vi "Tacking Helper - Jump Length.vi"(9 "Bounding box\nside length (m?)":dbl, 10 "Second\nArm Length":dbl, 11 "Starting\nArm Length":dbl) -> (3 "Jump Length (m)":dbl)   [LabVIEW 2011]
doc: "By taking the bounding box length and knowing that two right triangles are formed, the jump length made by one tack can be found."
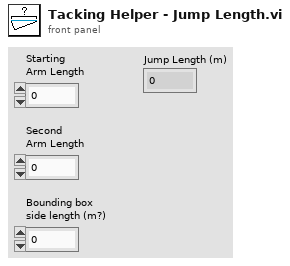
[diagram p1: front panel]
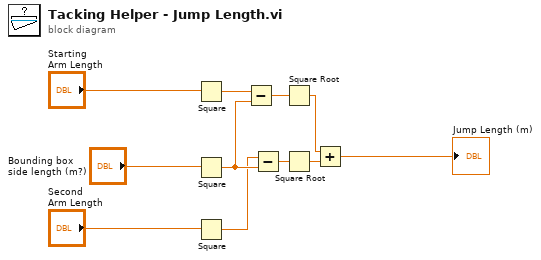
[diagram p0: block diagram]
diagram:
  n1 = Square(x="Starting\nArm Length") -> (x^2=w2:dbl)
  n2 = Square(x="Bounding box\nside length (m?)") -> (x^2=w4:dbl)
  n3 = Square(x="Second\nArm Length") -> (x^2=w3:dbl)
  n4 = Subtract(x=w2, y=w4) -> (x-y=w6:dbl)
  n5 = Subtract(x=w3, y=w4) -> (x-y=w5:dbl)
  n6 = Square Root(x=w6) -> (sqrt(x)=w7:dbl)
  n7 = Square Root(x=w5) -> (sqrt(x)=w8:dbl)
  n8 = Add(x=w7, y=w8) -> (x+y=→"Jump Length (m)":dbl)
